vi "Init Generic Message.vi"(5 "KVP Message":refnum<class "TestManagerMsg.KVP.lvclass">, 7 "overwrite?":bool=TRUE, 8 "value":variant, 9 "key":string, 10 "self-id":string, 11 "owner-id":string) -> (3 "Message":refnum<class "TestManagerMsg.lvclass">)   [LabVIEW 2013, in "Caraya.lvlib" / "TestManagerMsg.KVP.lvclass"]
uses:
  TestManagerMsg.KVP.lvclass
  Test Manager Message/TestManagerMsg.lvclass
  TestManagerMsg.KVP.lvclass/TestManagerMsg.KVP.ctl
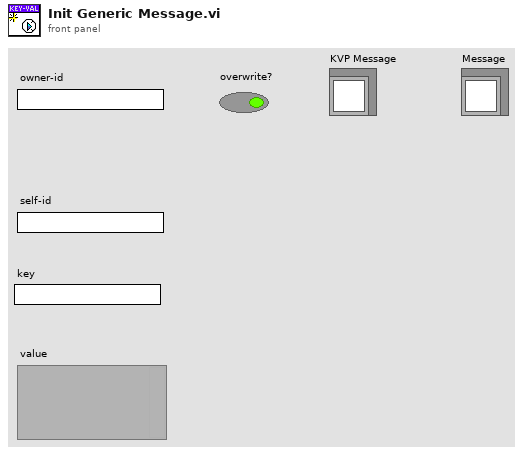
[diagram p1: front panel]
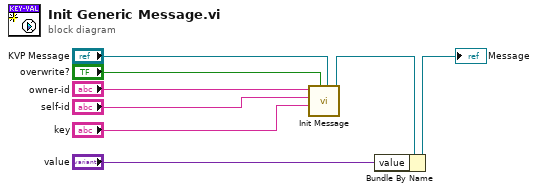
[diagram p0: block diagram]
diagram:
  n1 = call "Init Message.vi"("TestManagerMsg"="KVP Message", "overwrite?"="overwrite?", "key"="key", "self-id"="self-id", "owner-id"="owner-id") -> ("Message"=w6:refnum<class "TestManagerMsg.KVP.lvclass">)  [unwired: 6 in]
  n2 = Bundle By Name(cluster=w6, "value"="value") -> (→"Message":refnum<class "TestManagerMsg.KVP.lvclass">)
